vi "writeI8.vi"(8 "error in (no error)":errorcluster, 10 "Input":i8, 11 "ModbusBuffer in":refnum<class "ModbusBufferBuilder.lvclass">) -> (0 "error out":errorcluster, 3 "ModbusBuffer out":refnum<class "ModbusBufferBuilder.lvclass">)   [LabVIEW 2016, in "ModbusBufferBuilder.lvclass"]
uses:
  ModbusBufferBuilder.lvclass
  ModbusBufferBuilder.lvclass/ModbusBufferBuilder.ctl
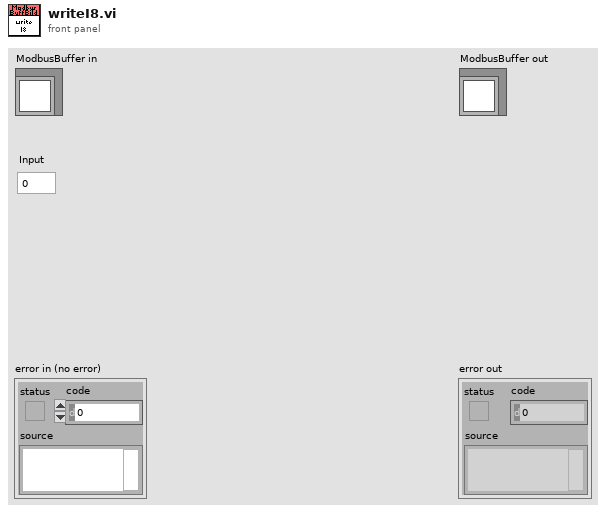
[diagram p1: front panel]
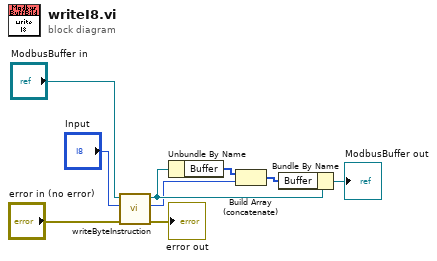
[diagram p0: block diagram]
diagram:
  n1 = call "writeByteInstruction.vi"("error in (no error)"="error in (no error)", "Input"="Input", "ModbusBuffer in"="ModbusBuffer in") -> ("error out"=→"error out":errorcluster, "Output"=w2:u16, "ModbusBuffer out"=w5:refnum<class "ModbusBufferBuilder.lvclass">)  [unwired: 6 in]
  n2 = Unbundle By Name(w5) -> ("Buffer"=w3:u16[])
  n3 = Build Array (concatenate)(w3, w2) -> (w1:u16[])
  n4 = Bundle By Name(cluster=w5, "Buffer"=w1) -> (→"ModbusBuffer out":refnum<class "ModbusBufferBuilder.lvclass">)
